vi "Key Store.vi"(1 "Key Store Actions (default Get Keys)":T2=enum."Get Keys") -> (0 "Key Store":T1)   [LabVIEW 2013]
uses:
  Controls/Key Store Actions.ctl
  Controls/JSON Key List.ctl
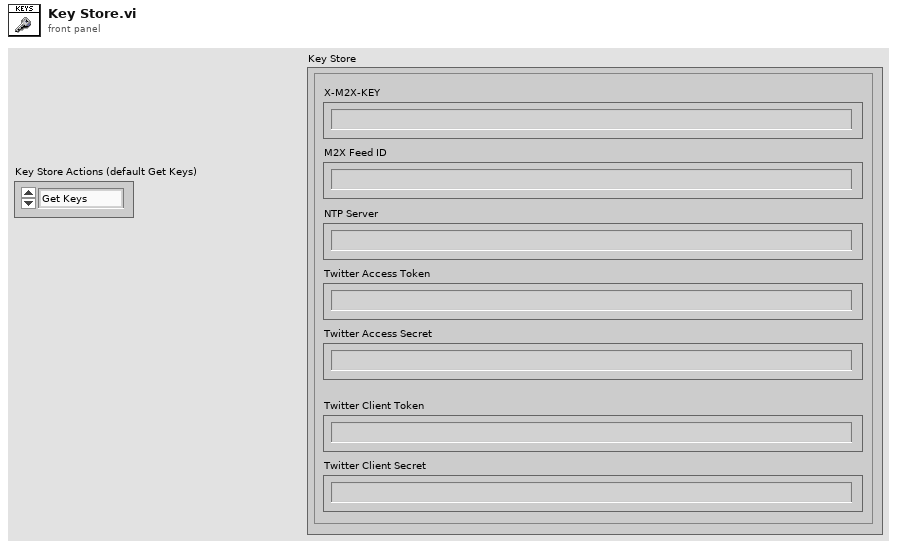
[diagram p1: front panel]
types:
  T1 = typedef "JSON Key List.ctl" = cluster{"X-M2X-KEY":string, "M2X Feed ID":string, "Twitter Access Token":string, "Twitter Access Secret":string, "Twitter Client Token":string, "Twitter Client Secret":string, "NTP Server":string}
  T2 = typedef "Key Store Actions.ctl" = enum16{"Load Keys File", "Get Keys", "Save Keys File"}
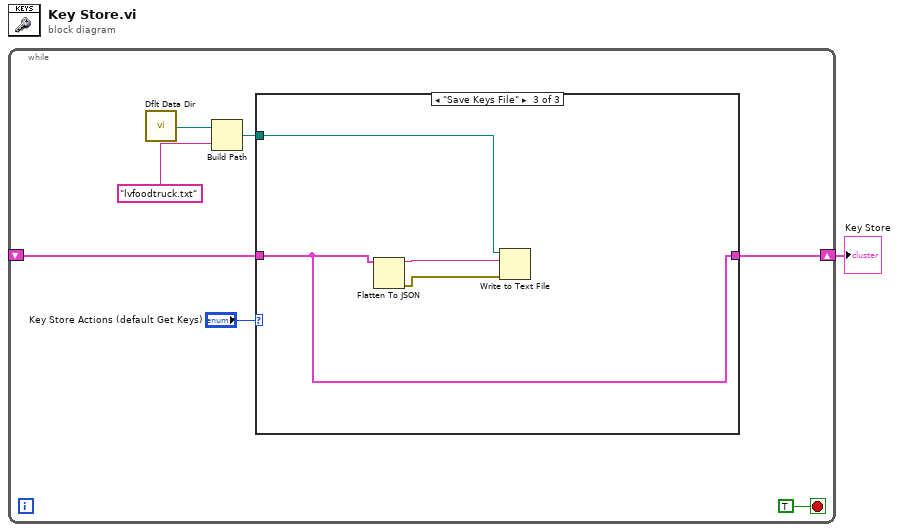
[diagram p0: block diagram]
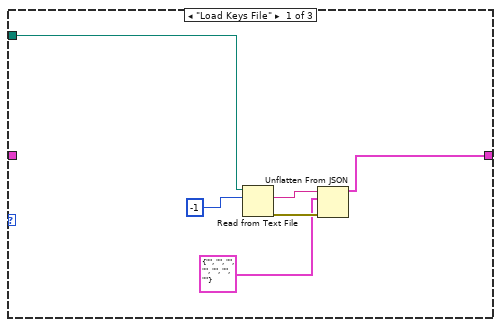
[diagram p2: hidden frame]
diagram:
  n1 = while {
    shift-right: [w7] -> w1
    shift-left: _ -> [w2]
    stop <- TRUE stop-if-true
    n2 = call <vilib>:"Dflt Data Dir.vi"() -> ("App:Default Data Directory"=w5:path)
    n3 = Build Path(base path=w5, name or relative path="lvfoodtruck.txt") -> (appended path=w4:path)
    n4 = case shown="\"Save Keys File\"" "Key Store Actions (default Get Keys)" {
      tunnel: [w10 w15 w16] -> w7
      tunnel: w4 -> [w9 _ w17]
      tunnel: w2 -> [_ w15 w16]
      frame "Load Keys File" {
        n5 = Read from Text File(file (use dialog)=w9, count=-1) -> (text=w13:string, error out=w12:errorcluster)  [unwired: 2 in, 2 out]
        n6 = Unflatten From JSON(JSON string=w13, type and defaults=T1 {"X-M2X-KEY"="", "M2X Feed ID"="", "Twitter Access Token"="", "Twitter Access Secret"="", "Twitter Client Token"="", "Twitter Client Secret"="", "NTP Server"=""} ("Key Store"), error in (no error)=w12) -> (value=w10:T1)  [unwired: 4 in, 1 out]
      }
      frame "Get Keys" {
      }
      frame "Save Keys File" {
        n7 = Flatten To JSON(anything=w16) -> (JSON string=w18:string, 11:w19:errorcluster)  [unwired: 2 in]
        n8 = Write to Text File(file (use dialog)=w17, text=w18, error in=w19) -> ()  [unwired: 1 in, 3 out]
      }
    }
  }
  "Key Store" <- w1
